vi "Raft_wars_Player_Board.vi"(11 "Player Ship Inputs":T1(array[cluster]) {"Y-Coordinate" min=0 max=7; "X-Coordinate" min=0 max=7}) -> (3 "Array":dbl[][](array[numeric]))   [LabVIEW 2026]
panel:
  in  "Emergency Stop":bool
  out "Game Status":string
  out "Ships Placed":dbl
  out "Losses":dbl
  out "Computer Hits":dbl
  out "Wins":dbl
  out "Player Hits":dbl
  in  "Attack":bool
  in  "Play Again":bool
  in  "Place Ship":bool
  in  "Attack Y":dbl
  in  "Attack X":dbl
  in  "Ship Y":i32
  in  "Ship X":i32
  out "Computer  Board":u32[][][][][][][][](array[colorbox])
  out "Player Board":u32[][][][][][][][](array[colorbox])
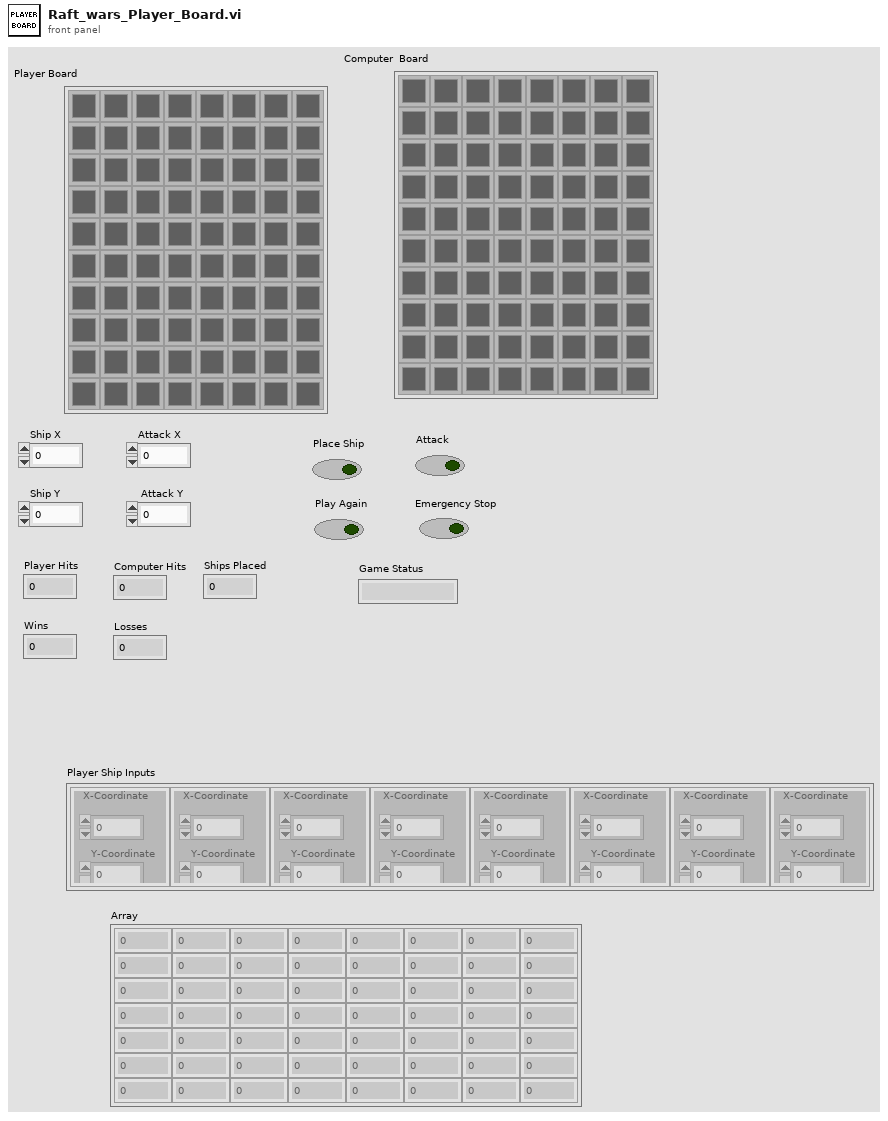
[diagram p1: front panel]
types:
  T1 = cluster{"X-Coordinate":i32, "Y-Coordinate":i32}[]
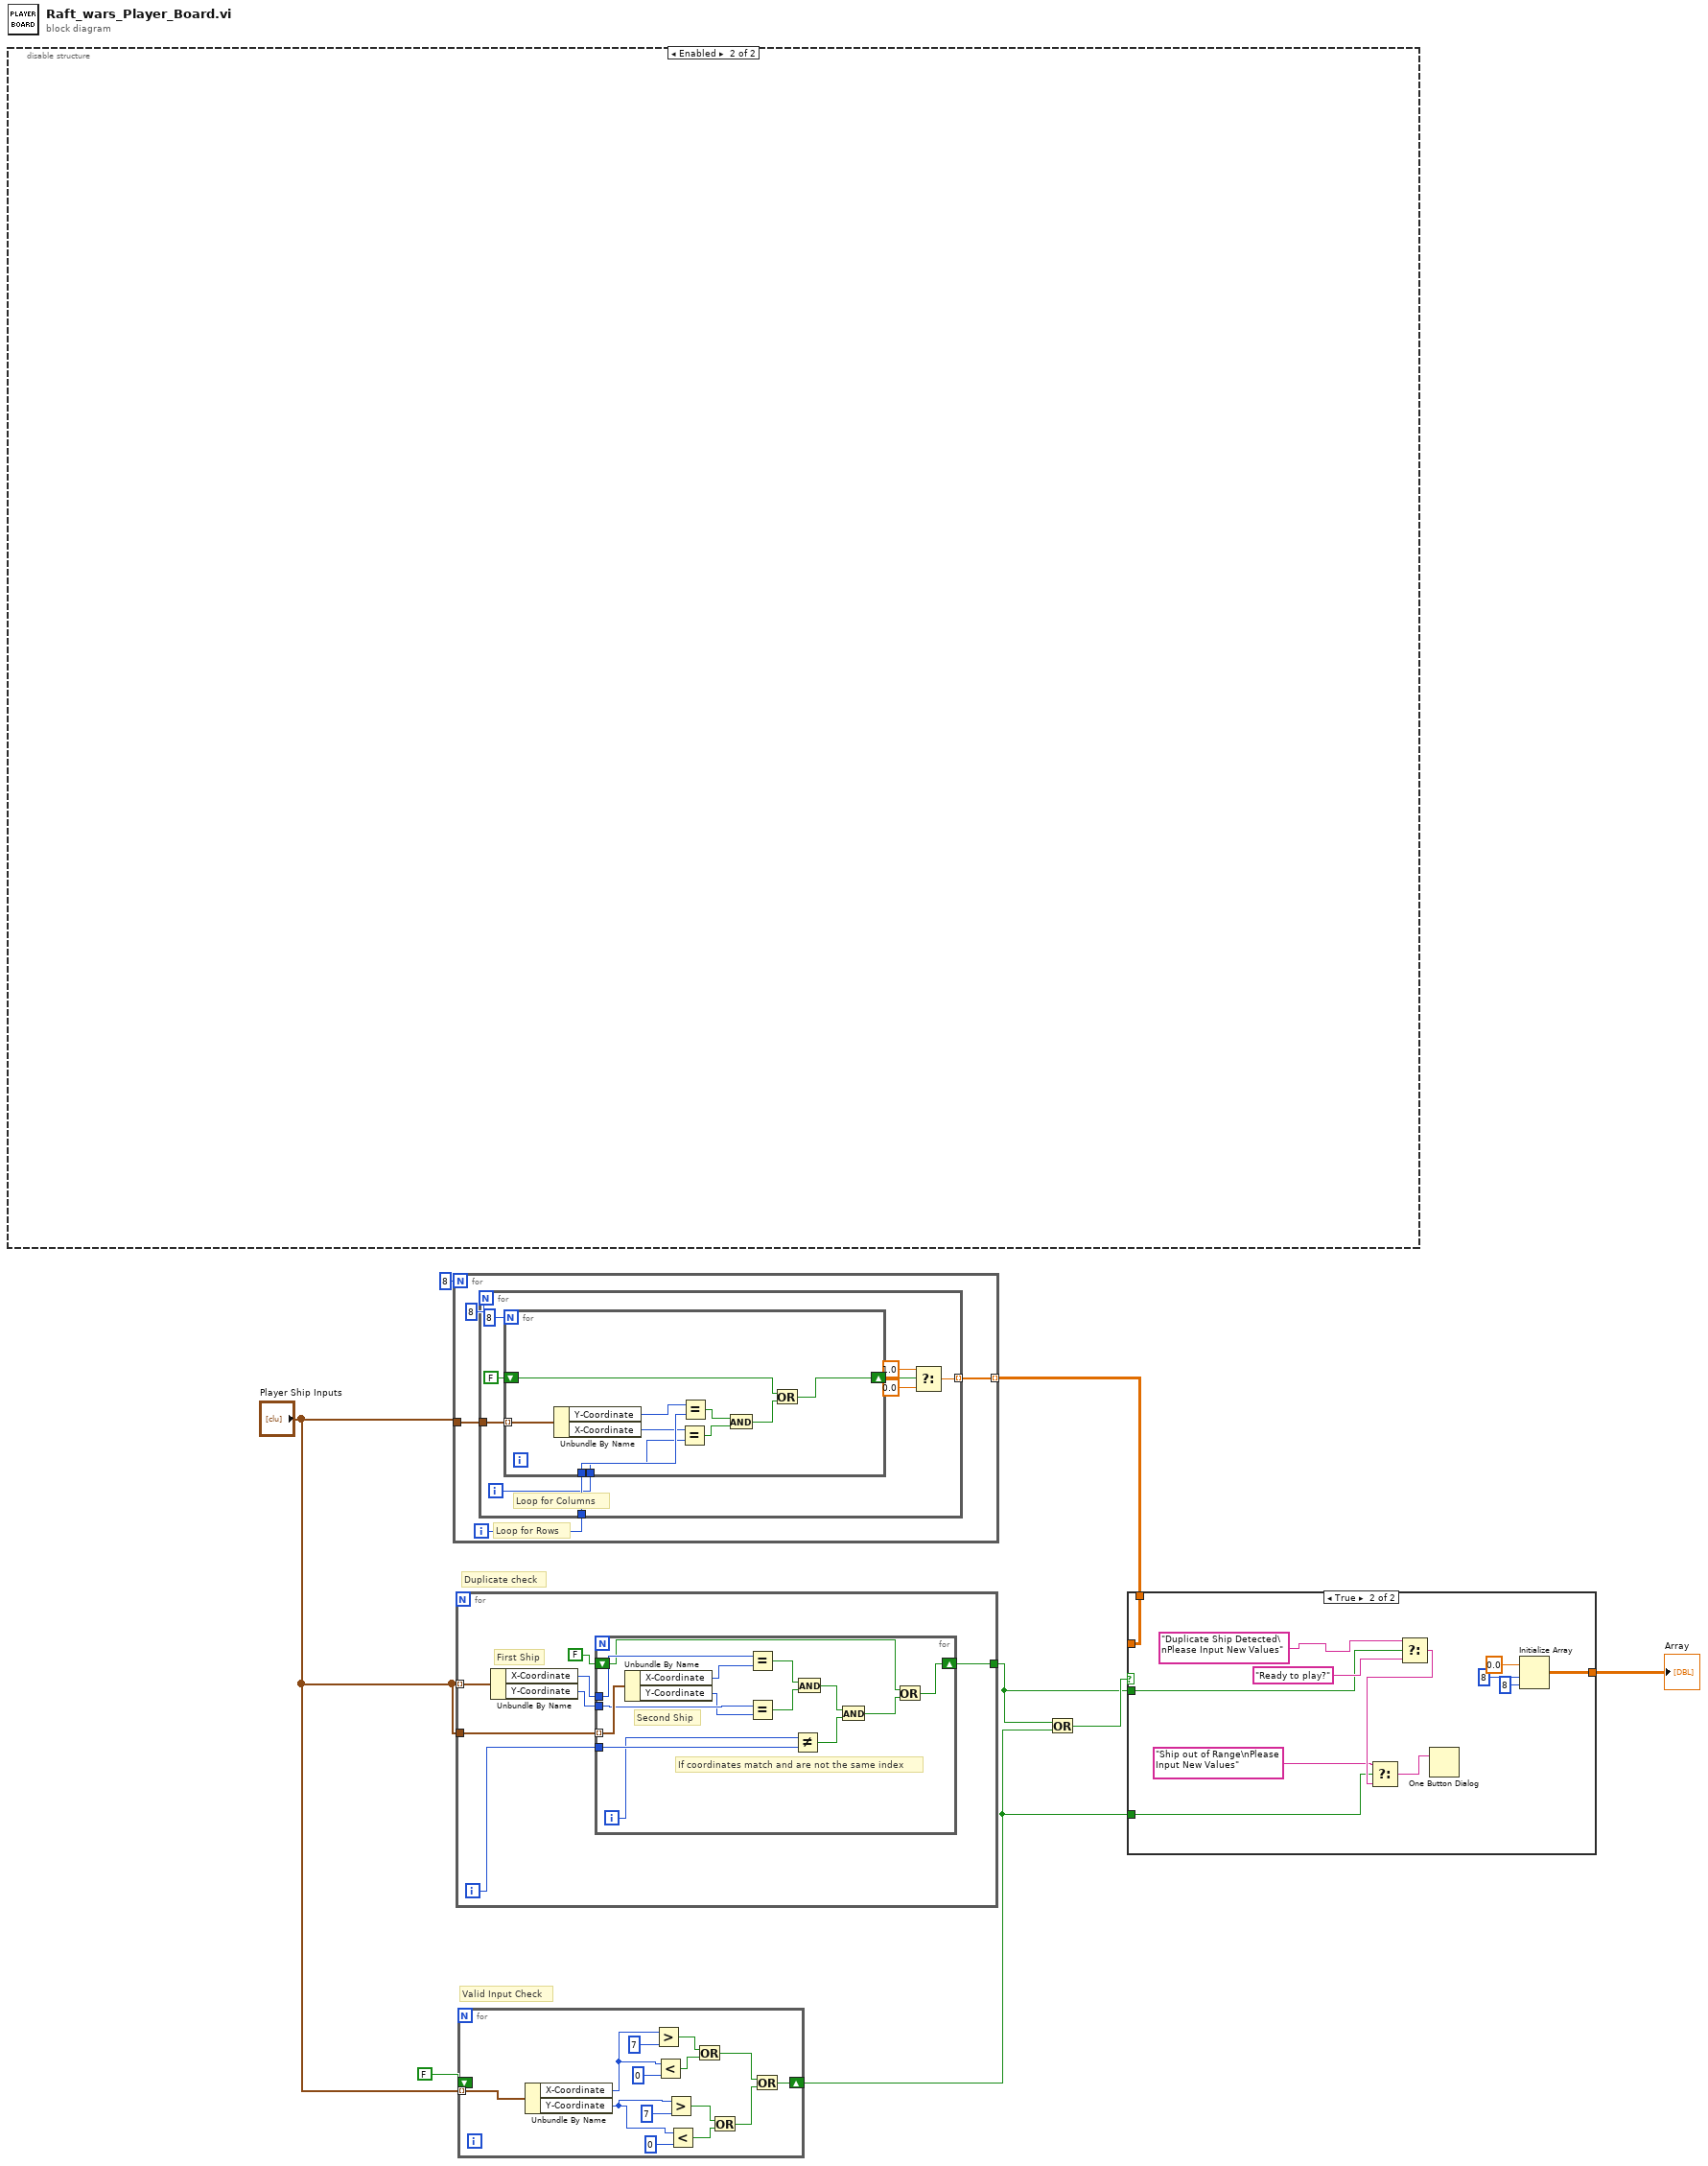
[diagram p0: block diagram]
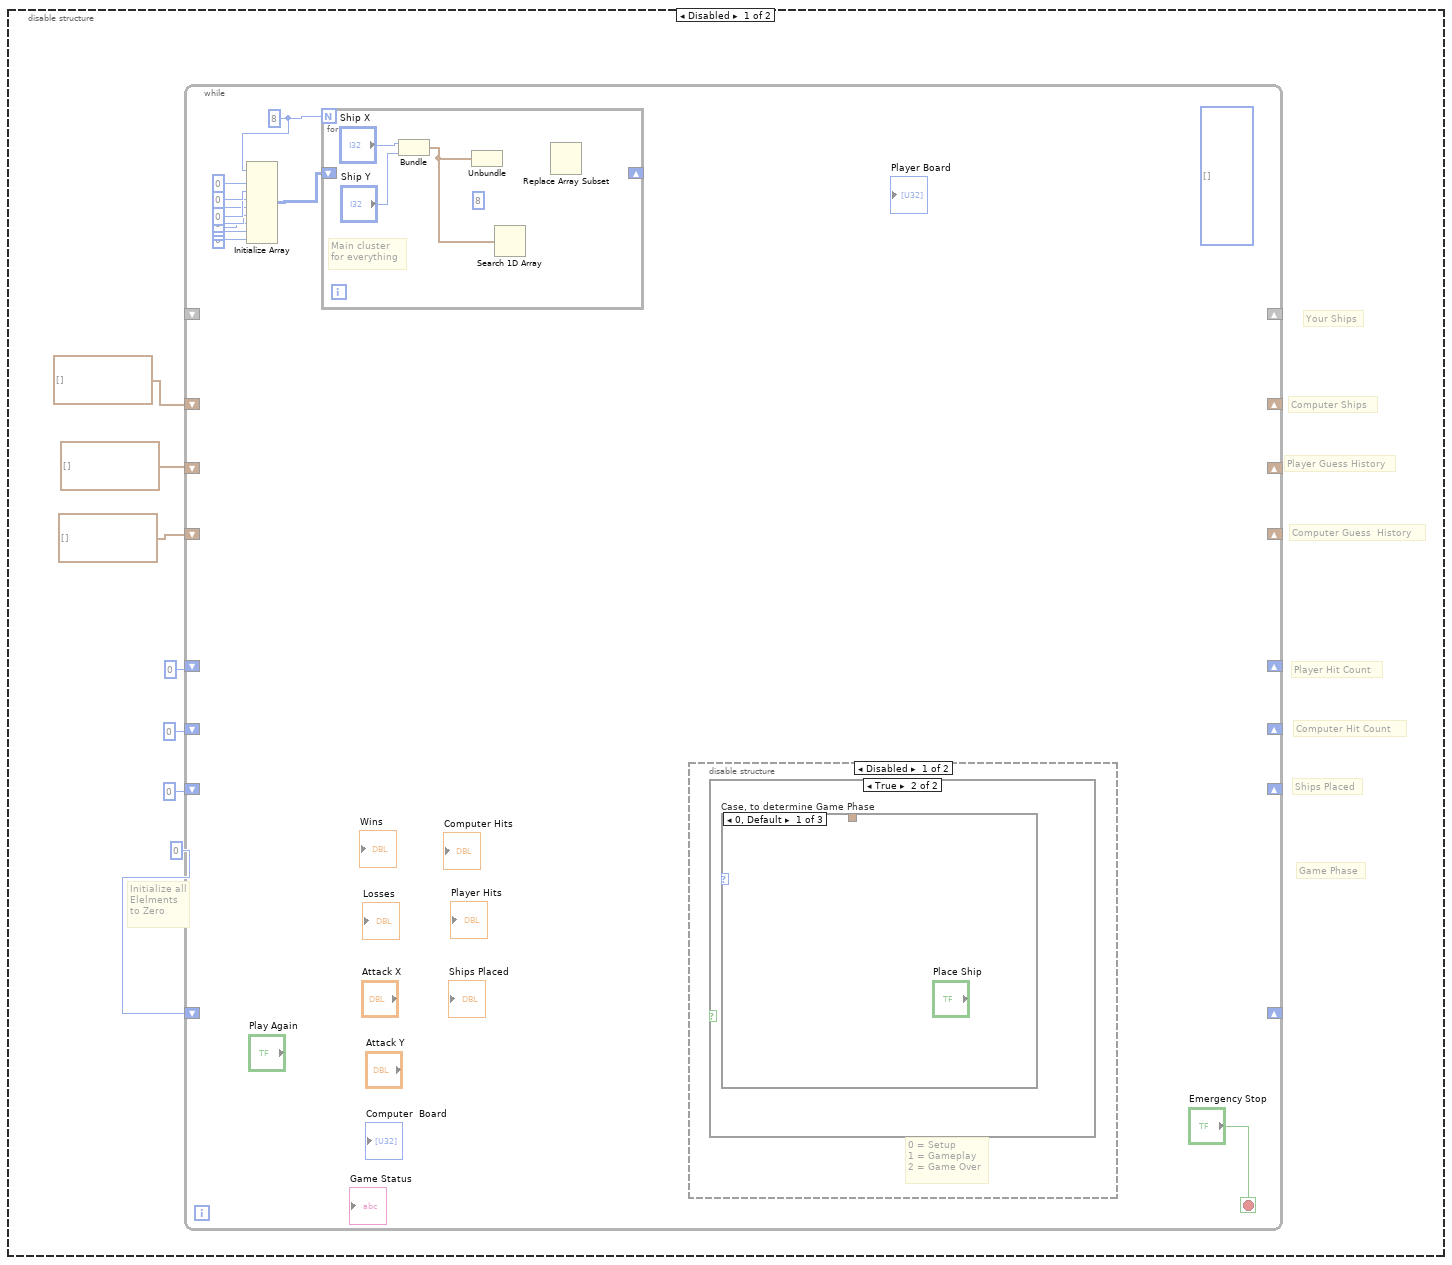
[diagram p3: hidden frame]
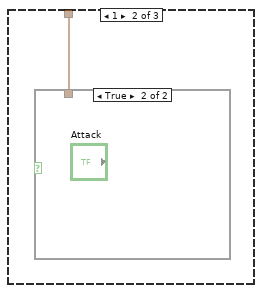
[diagram p5: hidden frame]
diagram:
  # "Valid Input Check"
  # "Duplicate check"
  n1 = disable-structure shown="Enabled" {
    frame Disabled {
      # "Initialize all\nElelments\nto Zero"
      # "Ships Placed"
      # "Your Ships"
      # "Computer Ships"
      # "Player Guess History"
      # "Computer Guess  History"
      # "Player Hit Count"
      # "Computer Hit Count"
      # "Game Phase"
      n2 = while {
        shift-right: _ -> [_]
        shift-left: _ -> [_]
        shift-right: _ -> [_]
        shift-left: cluster{dbl, dbl}[] [] -> [_]
        shift-right: _ -> [_]
        shift-left: cluster{dbl, dbl}[] [] -> [_]
        shift-right: _ -> [_]
        shift-left: cluster{dbl, dbl}[] [] -> [_]
        shift-right: _ -> [_]
        shift-left: 0 -> [_]
        shift-right: _ -> [_]
        shift-left: 0 -> [_]
        shift-right: _ -> [_]
        shift-left: 0 -> [_]
        shift-right: _ -> [_]
        shift-left: 0 -> [_]
        stop <- "Emergency Stop" stop-if-true
        w24 = 8
        (unwired) u32[][][][][][][][] [] ("PLayer 1 Board 2")
        n3 = Initialize Array(w24, 0 ("dimension size"), 0 ("dimension size"), 0 ("dimension size"), 0 ("dimension size"), 0 ("dimension size"), 0 ("dimension size"), 0 ("dimension size"), 0 ("dimension size")) -> (w25:i32[][][][][][][][])
        n4 = for {
          N: w24 -> [_]
          shift-right: _ -> [w27]
          shift-left: w25 -> [_]
          (unwired) 8
          # "Main cluster\nfor everything"
          n5 = Bundle("Ship X"="Ship X", "Ship Y"="Ship Y") -> (w28:cluster{"Ship X":i32, "Ship Y":i32})  [unwired: 1 in]
          n6 = Unbundle(w28) -> ()  [unwired: 2 out]
          n7 = Search 1D Array(element=w28) -> ()  [unwired: 2 in, 1 out]
          n8 = Replace Array Subset() -> ()  [unwired: 3 in, 1 out]
        }
        n9 = disable-structure shown="Disabled" {
          frame Disabled {
            # "0 = Setup\n1 = Gameplay\n2 = Game Over"
            n10 = case shown="True" {
              selector: _ -> [_ _]
              frame False {
              }
              frame True {
                n11 = case "Case, to determine Game Phase" shown="0, Default" {
                  selector: _ -> [_ _ _]
                  tunnel: _ -> [_ w31 _]
                  frame 0, Default {
                  }
                  frame 1 {
                    n12 = case shown="True" {
                      selector: _ -> [_ _]
                      tunnel: w31 -> [_ _]
                      frame False {
                      }
                      frame True {
                      }
                    }
                  }
                  frame 2 {
                  }
                }
              }
            }
          }
          frame Enabled {
          }
        }
      }
    }
    frame Enabled {
    }
  }
  n13 = for {
    N: 8 -> [_]
    tunnel: "Player Ship Inputs" -> [w32]
    tunnel: [w33] -> w5 mode=indexing
    i -> [w34]
    # "Loop for Rows"
    n14 = for {
      N: 8 -> [_]
      tunnel: w34 -> [w44]
      tunnel: [w39] -> w33 mode=indexing
      tunnel: w32 -> [w36]
      i -> [w43]
      # "Loop for Columns"
      n15 = for {
        N: 8 -> [_]
        tunnel: w44 -> [w48]
        tunnel: w43 -> [w47]
        shift-right: [w49] -> w42
        shift-left: FALSE -> [w50]
        tunnel: w36 -> [w46] mode=indexing
        n16 = Unbundle By Name(w46) -> ("Y-Coordinate"=w54:i32, "X-Coordinate"=w45:i32)
        n17 = Equal?(x=w45, y=w47) -> (x = y?=w52:bool)
        n18 = Equal?(x=w54, y=w48) -> (x = y?=w53:bool)
        n19 = And(x=w53, y=w52) -> (x .and. y?=w51:bool)
        n20 = Or(x=w50, y=w51) -> (x .or. y?=w49:bool)
      }
      n21 = Select(t=1.0, s=w42, f=0.0) -> (s? t:f=w39:dbl)
    }
  }
  n22 = for {
    tunnel: "Player Ship Inputs" -> [w57] mode=indexing
    tunnel: "Player Ship Inputs" -> [w56]
    tunnel: [w55] -> w1
    i -> [w59]
    # "First Ship"
    n23 = Unbundle By Name(w57) -> ("X-Coordinate"=w61:i32, "Y-Coordinate"=w60:i32)
    n24 = for {
      tunnel: w56 -> [w75] mode=indexing
      tunnel: w61 -> [w74]
      tunnel: w60 -> [w72]
      tunnel: w59 -> [w68]
      shift-right: [w62] -> w55
      shift-left: FALSE -> [w64]
      i -> [w67]
      # "If coordinates match and are not the same index"
      # "Second Ship"
      n25 = Unbundle By Name(w75) -> ("X-Coordinate"=w73:i32, "Y-Coordinate"=w71:i32)
      n26 = Equal?(x=w74, y=w73) -> (x = y?=w69:bool)
      n27 = Equal?(x=w72, y=w71) -> (x = y?=w70:bool)
      n28 = Not Equal?(x=w67, y=w68) -> (x != y?=w65:bool)
      n29 = And(x=w69, y=w70) -> (x .and. y?=w66:bool)
      n30 = And(x=w66, y=w65) -> (x .and. y?=w63:bool)
      n31 = Or(x=w64, y=w63) -> (x .or. y?=w62:bool)
    }
  }
  n32 = for {
    tunnel: "Player Ship Inputs" -> [w89] mode=indexing
    shift-right: [w76] -> w2
    shift-left: FALSE -> [_]
    n33 = Unbundle By Name(w89) -> ("X-Coordinate"=w86:i32, "Y-Coordinate"=w83:i32)
    n34 = Greater?(x=w86, y=7) -> (0:w81:bool)
    n35 = Less?(x=w86, y=0) -> (x < y?=w82:bool)
    n36 = Greater?(x=w83, y=7) -> (0:w80:bool)
    n37 = Less?(x=w83, y=0) -> (x < y?=w79:bool)
    n38 = Or(x=w81, y=w82) -> (x .or. y?=w78:bool)
    n39 = Or(x=w80, y=w79) -> (x .or. y?=w77:bool)
    n40 = Or(x=w78, y=w77) -> (x .or. y?=w76:bool)
  }
  n41 = Or(x=w1, y=w2) -> (x .or. y?=w3:bool)
  n42 = case shown="True" w3 {
    tunnel: [w90 w101] -> w4
    tunnel: [_ w99] -> _
    tunnel: w5 -> [w90 w99]
    tunnel: w2 -> [_ w92]
    tunnel: w1 -> [_ w91]
    frame False {
    }
    frame True {
      n43 = Select(t="Duplicate Ship Detected\nPlease Input New Values", s=w91, f="Ready to play?") -> (s? t:f=w97:string)
      n44 = Select(t="Ship out of Range\nPlease Input New Values", s=w92, f=w97) -> (s? t:f=w95:string)
      n45 = One Button Dialog(message=w95) -> ()  [unwired: 1 in, 1 out]
      n46 = Initialize Array(0.0 ("element"), 8 ("dimension size"), 8 ("dimension size")) -> (w101:dbl[][])
    }
  }
  "Array" <- w4
